vi "6-3 hp34401 beep.vi"(1 "Delay (s)":dbl=2.0 format="%.2f", 2 "n° beep":u32) -> (0 "error out":bool)   [LabVIEW 2012]
panel:
  in  "addr":string="4"
  # "1. TEST INVIO COMANDI\n    Realizzare un VI che, nella sua versione iniziale, invia un BEEP allo strumento; nella versione finale il VI dovrˆ\n    far s“ che lo strumento emetta un determinato numero di BEEP consecutivi (selezionati tramite un controllo da pannello) \n    ogni 2 secondi. In caso di errore il ritardo di 2 secondi dovrˆ essere annullato, il VI dovrˆ terminare e un indicatore \n    booleano segnalerˆ tale condizione."
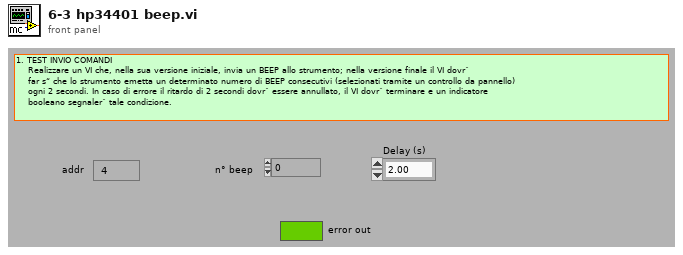
[diagram p1: front panel]
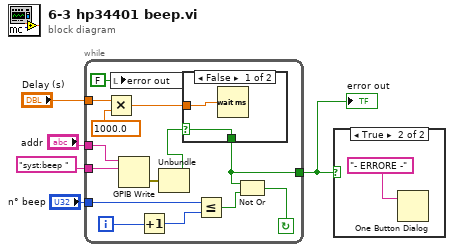
[diagram p0: block diagram]
diagram:
  n1 = while {
    tunnel: "syst:beep " -> [w14]
    tunnel: "addr" -> [w15]
    tunnel: "Delay (s)" -> [w13]
    tunnel: "n° beep" -> [w10]
    tunnel: [w7] -> w1
    i -> [w19]
    stop <- w16 continue-if-true
    n2 = Multiply(x=w13, y=1000.0) -> (x*y=w9:dbl)
    n3 = local write "error out"(FALSE ("error out")) -> ()
    n4 = GPIB Write(0:w15, 1:w14) -> (6:w11:errorcluster)  [unwired: 3 in, 1 out]
    n5 = Increment(x=w19) -> (x+1=w18:i32)
    n6 = Unbundle(w11) -> ("status"=w8:bool)  [unwired: 2 out]
    n7 = case shown="False" w8 {
      selector: w8 -> [w20 w22]
      tunnel: w9 -> [w21 _]
      tunnel: [w20 w22] -> w7
      frame False {
        n8 = Wait (ms)(milliseconds to wait=w21) -> ()  [unwired: 1 out]
      }
      frame True {
      }
    }
    n9 = Less Or Equal?(x=w10, y=w18) -> (x <= y?=w17:bool)
    n10 = Not Or(1:w17, 2:w7) -> (0:w16:bool)
  }
  "error out" <- w1
  n11 = case shown="True" w1 {
    frame False {
    }
    frame True {
      n12 = One Button Dialog(message="- ERRORE -") -> ()  [unwired: 1 in, 1 out]
    }
  }
